vi "Delete Dir.vi"(8 "error in (no error)":errorcluster, 11 "dup path":path) -> (0 "error out":errorcluster, 3 "deleted path":path)   [LabVIEW 2014, in "lvprj2html.lvlib"]
uses:
  lvprj2html.lvlib
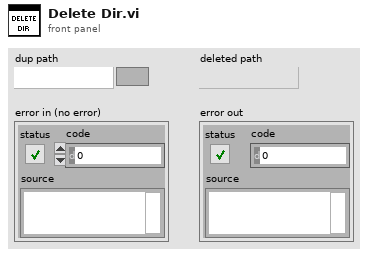
[diagram p1: front panel]
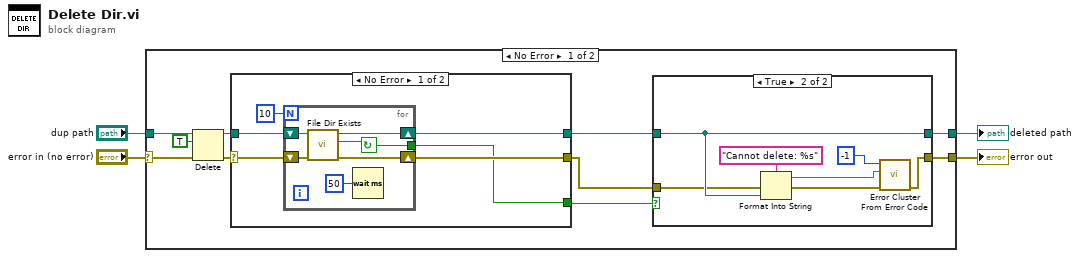
[diagram p0: block diagram]
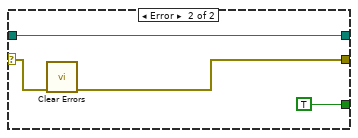
[diagram p3: hidden frame]
diagram:
  n1 = case shown="No Error" "error in (no error)" {
    selector: "error in (no error)" -> [w12 w40]
    tunnel: [w5 w40] -> w4
    tunnel: [w7 w41] -> w3
    tunnel: "dup path" -> [w13 w41]
    frame No Error {
      n2 = Delete(path (use dialog)=w13, entire hierarchy (F)=TRUE, error in=w12) -> (deleted path=w11:path, error out=w10:errorcluster)  [unwired: 2 in, 1 out]
      n3 = case shown="No Error" w10 {
        selector: w10 -> [w28 w38]
        tunnel: w11 -> [w29 w39]
        tunnel: [w26 w39] -> w8
        tunnel: [w25 w36] -> w6
        tunnel: [w24 TRUE] -> w9
        frame No Error {
          n4 = for {
            N: 10 -> [_]
            shift-right: [w31] -> w26
            shift-left: w29 -> [w32]
            shift-right: [w33] -> w25
            shift-left: w28 -> [w34]
            tunnel: [w30] -> w24
            stop <- w30 continue-if-true
            n5 = call "File Dir Exists.vi"("error in (no error)"=w34, "path"=w32) -> ("error out"=w33:errorcluster, "exists"=w30:bool, "path out"=w31:path)  [unwired: 7 in]
            n6 = Wait (ms)(milliseconds to wait=u32 50) -> ()  [unwired: 1 out]
          }
        }
        frame Error {
          n7 = call <vilib>:"Clear Errors.vi"("error in (no error)"=w38) -> ("error out"=w36:errorcluster)  [unwired: 5 in, 1 out]
        }
      }
      n8 = case shown="True" w9 {
        tunnel: w8 -> [w15 w19]
        tunnel: [w15 w19] -> w7
        tunnel: w6 -> [w16 w18]
        tunnel: [w16 w17] -> w5
        frame False {
        }
        frame True {
          n9 = Format Into String(format string="Cannot delete: %s", error in=w18, w19) -> (resulting string=w22:string, error out=w23:errorcluster)  [unwired: 1 in]
          n10 = call <vilib>:"Error Cluster From Error Code.vi"("error in (no error)"=w23, "error message (\"\")"=w22, "error code (0)"=-1) -> ("error out"=w17:errorcluster)  [unwired: 6 in]
        }
      }
    }
    frame Error {
    }
  }
  "error out" <- w4
  "deleted path" <- w3
